vi "Connect.vi"(6 "Timeout(ms)":i32=1000, 8 "error in (no error)":errorcluster, 11 "NetworkConnection in":refnum<class "NetworkConnection.lvclass">) -> (0 "error out":errorcluster, 2 "Connected?":bool, 3 "NetworkConnection out":refnum<class "NetworkConnection.lvclass">)   [LabVIEW 2020, in "NetworkConnection.lvclass"]
doc: "Tries to connect for the desired timeout period. If the connection is successful, the Connected? output will return TRUE.\nJKI Network Streams Connection 1.1.1.15\nJavier Ruiz - JKI\nCopyright (c) 2020, JKI\n\nThis library is provided \"AS IS\" ,WITHOUT WARRANTIES OR CONDITIONS OF ANY KIND, either express or implied."
uses:
  NetworkConnection.lvclass
  NetworkMessage--Cluster.ctl
  NetworkCommand--Cluster.ctl
  NetworkConnection.lvclass/NetworkConnection.ctl
panel:
  # "Copyright © 2020 JKI All rights reserved.\n\nAuthor: Javier Ruiz <javier.ruiz@jki.net>\n\nThis library is provided \"AS IS\" ,WITHOUT WARRANTIES OR \nCONDITIONS OF ANY KIND, either expressed or implied.\n\nJKI -- jki.net"
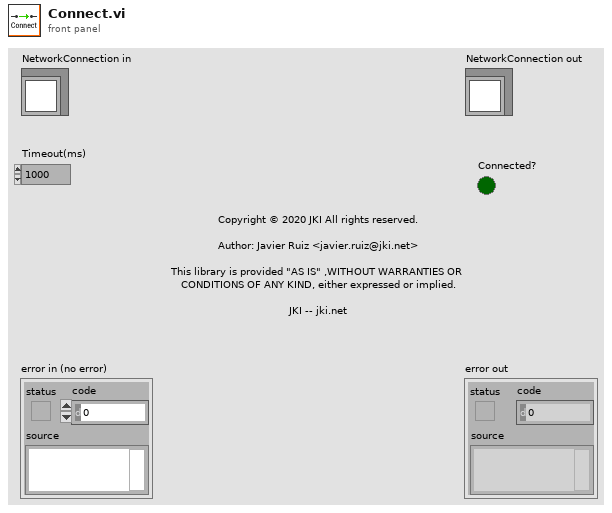
[diagram p1: front panel]
types:
  T1 = typedef "NetworkConnection.lvclass/NetworkMessage--Cluster.ctl" = cluster{"NetworkCommand":T2, "Wait for Ack?":bool, "Ack Id":i32}
  T2 = typedef "NetworkConnection.lvclass/NetworkCommand--Cluster.ctl" = cluster{"Command":string, "Arguments":variant, " Msg Id":i32}
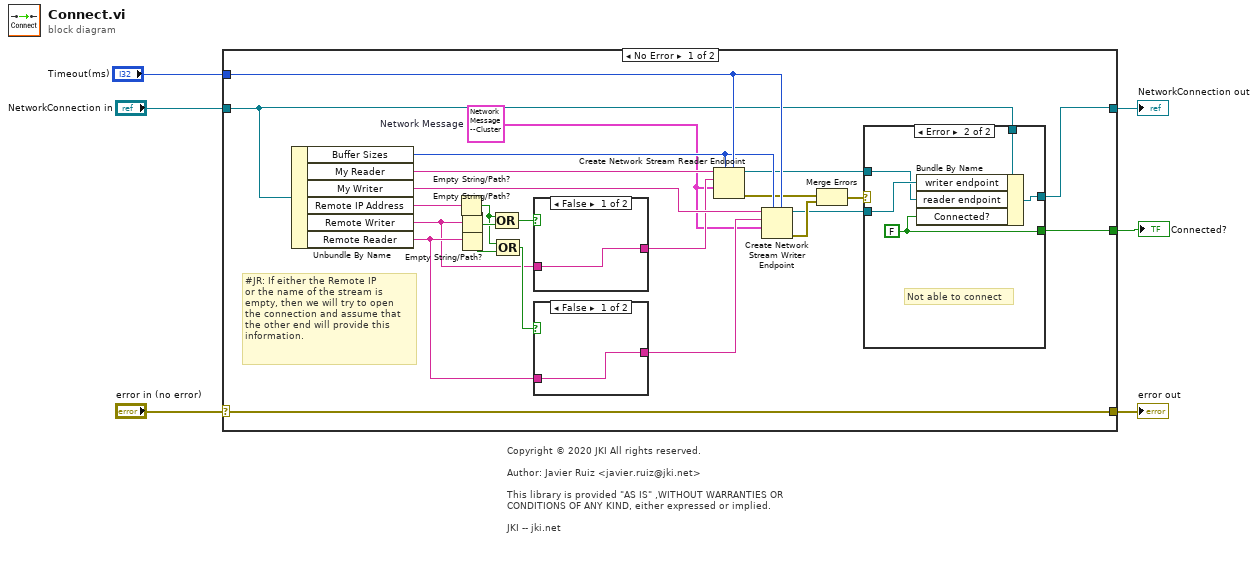
[diagram p0: block diagram]
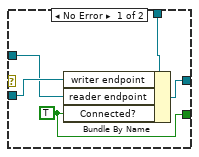
[diagram p2: hidden frame]
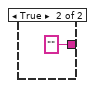
[diagram p3: hidden frame]
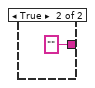
[diagram p4: hidden frame]
diagram:
  # "Copyright © 2020 JKI All rights reserved.\n\nAuthor: Javier Ruiz <javier.ruiz@jki.net>\n\nThis library is provided \"AS IS\" ,WITHOUT WARRANTIES OR \nCONDITIONS OF ANY KIND, either expressed or implied.\n\nJKI -- jki.net"
  n1 = case shown="No Error" "error in (no error)" {
    selector: "error in (no error)" -> [w29 w46]
    tunnel: [w29 w46] -> w5
    tunnel: [w12 w45] -> w3
    tunnel: "NetworkConnection in" -> [w13 w45]
    tunnel: "Timeout(ms)" -> [w18 _]
    tunnel: [w11 _] -> w1
    frame No Error {
      w8 = T1 {"NetworkCommand"={"Command"="", "Arguments"=variant, " Msg Id"=0}, "Wait for Ack?"=FALSE, "Ack Id"=0}  # Network Message
      # "#JR: If either the Remote IP\nor the name of the stream is\nempty, then we will try to open\nthe connection and assume that\nthe other end will provide this\ninformation."
      n2 = Unbundle By Name(w13) -> ("Buffer Sizes"=w17:i32, "My Reader"=w30:string, "My Writer"=w28:string, "Remote IP Address"=w22:string, "Remote Writer"=w7:string, "Remote Reader"=w21:string)
      n3 = Empty String/Path?(string/path=w22) -> (empty?=w25:bool)
      n4 = Empty String/Path?(string/path=w7) -> (empty?=w27:bool)
      n5 = Empty String/Path?(string/path=w21) -> (empty?=w24:bool)
      n6 = Compound Arithmetic op=OR(w25, w27) -> (w26:bool)
      n7 = Compound Arithmetic op=OR(w25, w24) -> (w23:bool)
      n8 = case shown="False" w26 {
        tunnel: w7 -> [w43 _]
        tunnel: [w43 ""] -> w20
        frame False {
        }
        frame True {
        }
      }
      n9 = case shown="False" w23 {
        tunnel: w21 -> [w41 _]
        tunnel: [w41 ""] -> w19
        frame False {
        }
        frame True {
        }
      }
      n10 = Create Network Stream Reader Endpoint(5:w18, 7:w17, 9:w8, 10:w20, 11:w30) -> (0:w16:errorcluster, 3:w10:refnum<k21>)  [unwired: 2 in]
      n11 = Create Network Stream Writer Endpoint(5:w18, 7:w17, 9:w8, 10:w19, 11:w28) -> (0:w15:errorcluster, 3:w9:refnum<k21>)  [unwired: 2 in]
      n12 = Merge Errors(w16, w15) -> (w14:errorcluster)
      n13 = case shown="Error" w14 {
        tunnel: w13 -> [w35 w40]
        tunnel: [w34 w39] -> w12
        tunnel: [w33 w38] -> w11
        tunnel: w10 -> [w31 w36]
        tunnel: w9 -> [w32 w37]
        frame No Error {
          w33 = TRUE ("Connected?")
          n14 = Bundle By Name(cluster=w35, "writer endpoint"=w32, "reader endpoint"=w31, "Connected?"=w33) -> (w34:refnum<class "NetworkConnection.lvclass">)
        }
        frame Error {
          w38 = FALSE ("Connected?")
          # "Not able to connect"
          n15 = Bundle By Name(cluster=w40, "writer endpoint"=w37, "reader endpoint"=w36, "Connected?"=w38) -> (w39:refnum<class "NetworkConnection.lvclass">)
        }
      }
    }
    frame Error {
    }
  }
  "error out" <- w5
  "NetworkConnection out" <- w3
  "Connected?" <- w1
